vi "Read MERCANCIA.vi"(8 "error in (no error)":errorcluster, 11 "BD_CAFÉ_MXN_ENG in":refnum<class "BD_CAFÉ_MXN_ENG.lvclass">) -> (0 "error out":errorcluster, 2 "MERCANCIA":refnum<vi>, 3 "BD_CAFÉ_MXN_ENG out":refnum<class "BD_CAFÉ_MXN_ENG.lvclass">)   [LabVIEW 2019, in "BD_CAFÉ_MXN_ENG.lvlib" / "BD_CAFÉ_MXN_ENG.lvclass"]
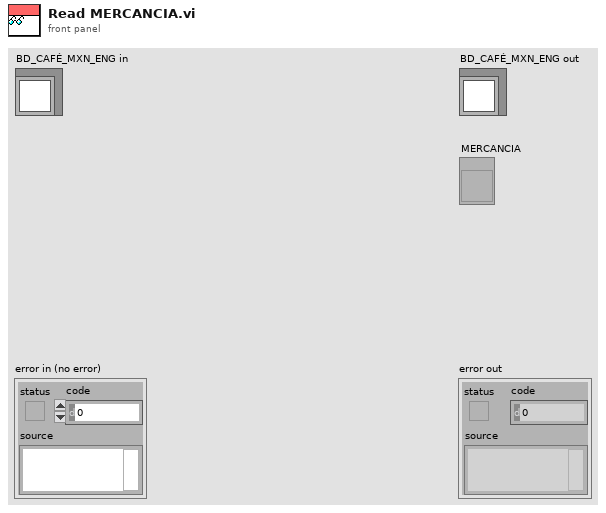
[diagram p1: front panel]
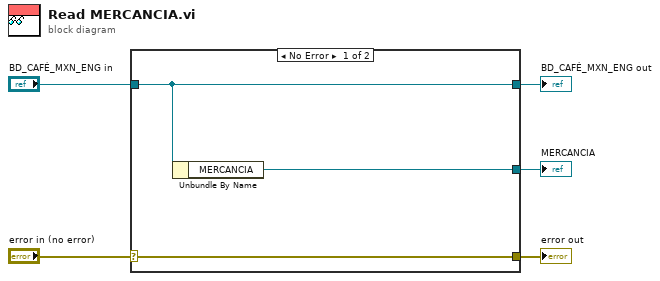
[diagram p0: block diagram]
diagram:
  n1 = case shown="No Error" "error in (no error)" {
    selector: "error in (no error)" -> [w8 w9]
    tunnel: [w8 w9] -> w4
    tunnel: [w7 w10] -> w2
    tunnel: "BD_CAFÉ_MXN_ENG in" -> [w7 w10]
    tunnel: [w6 _] -> w1
    frame No Error {
      n2 = Unbundle By Name(w7) -> ("MERCANCIA"=w6:refnum<vi>)
    }
    frame Error {
    }
  }
  "error out" <- w4
  "BD_CAFÉ_MXN_ENG out" <- w2
  "MERCANCIA" <- w1
